vi "dfd_Analysis Bank Build Output Waveform.vi"(6 "initH":bool, 7 "t0":timestamp, 8 "error in (no error)":errorcluster, 10 "y":dbl[][](array[numeric]), 11 "waveform in":waveform(dbl)={"t0"=timestamp(0 s since 1904-01-01), "dt"=0.0, "Y"=[]}) -> (0 "error out":errorcluster, 3 "y":waveform(dbl)[](array[waveform]), 5 "tf":timestamp)   [LabVIEW 2017, in "NI_DigFilter_FilterBank.lvlib"]
uses:
  <vilib>/addons/Digital Filter Design/NI_DigFilter_FilterBank.lvlib
  <vilib>/addons/Digital Filter Design/NI_DigFilterLicensed.lvlib
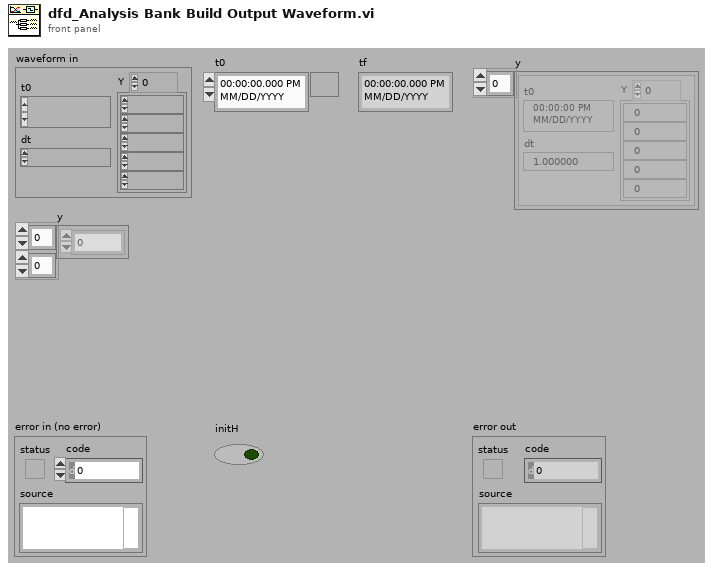
[diagram p1: front panel]
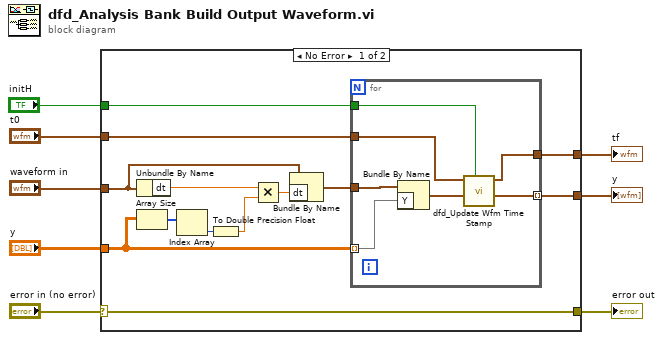
[diagram p0: block diagram]
diagram:
  n1 = case shown="No Error" "error in (no error)" {
    selector: "error in (no error)" -> [w13 w30]
    tunnel: "waveform in" -> [w19 _]
    tunnel: [w17 _] -> w7
    tunnel: "y" -> [w16 _]
    tunnel: [w13 w30] -> w5
    tunnel: "initH" -> [w12 _]
    tunnel: "t0" -> [w11 w29]
    tunnel: [w10 w29] -> w1
    frame No Error {
      n2 = Unbundle By Name(w19) -> ("dt"=w21:dbl)
      n3 = Array Size(array=w16) -> (size(s)=w15:i32[])
      n4 = Index Array(array=w15) -> (element=w14:i32)  [unwired: 1 in]
      n5 = To Double Precision Float(number=w14) -> (double precision float=w9:dbl)
      n6 = Multiply(x=w21, y=w9) -> (x*y=w20:dbl)
      n7 = Bundle By Name(cluster=w19, "dt"=w20) -> (w18:waveform(dbl))
      n8 = for {
        tunnel: w16 -> [w27] mode=indexing
        tunnel: w18 -> [w28]
        tunnel: [w24] -> w17 mode=indexing
        tunnel: w12 -> [w25]
        tunnel: w11 -> [w23]
        tunnel: [w22] -> w10
        n9 = Bundle By Name(cluster=w28, "Y"=w27) -> (w26:waveform(dbl))
        n10 = call <vilib>:"dfd_Update Wfm Time Stamp.vi"("init? (F)"=w25, "signal in"=w26, "t0"=w23) -> ("signal out"=w24:waveform(dbl), "tf"=w22:timestamp)  [unwired: 1 in, 6 out]
      }
    }
    frame Error {
    }
  }
  "y" <- w7
  "error out" <- w5
  "tf" <- w1
